vi "_emi_Loop Control single.vi"(0 "Loop ID in":u16, 7 "Enable":bool, 11 "error in (no error)":errorcluster) -> (4 "Loop ID out":u16, 15 "error out":errorcluster)   [LabVIEW 2011]
uses:
  _emi_Loop control int action.ctl
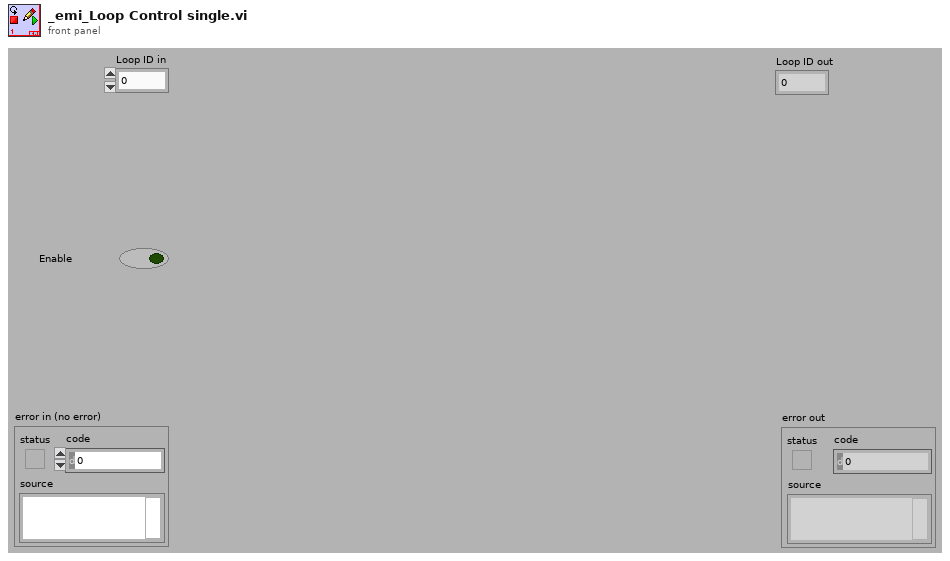
[diagram p1: front panel]
types:
  T1 = typedef "_emi_Loop control int action.ctl" = enum16{"Init index", "Get index", "Set index", "Get Size"}
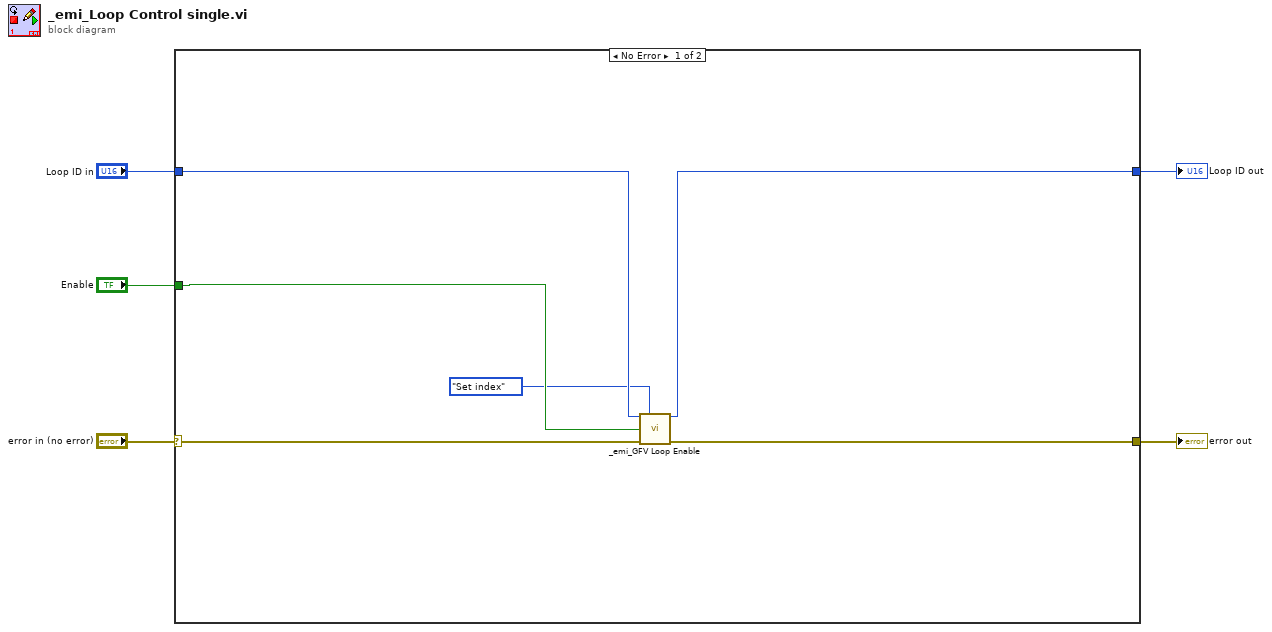
[diagram p0: block diagram]
diagram:
  n1 = case shown="No Error" "error in (no error)" {
    selector: "error in (no error)" -> [w11 w13]
    tunnel: [w10 w13] -> w4
    tunnel: [w8 w12] -> w3
    tunnel: "Loop ID in" -> [w9 w12]
    tunnel: "Enable" -> [w7 _]
    frame No Error {
      n2 = call "_emi_GFV Loop Enable.vi"("Loop Index/Numb"=w9, "Action(Get Index)"=_emi_Loop_control_int_action."Set index", "Loop enable In(T)"=w7, "error in (no error)"=w11) -> ("Index out"=w8:u16, "error out"=w10:errorcluster)  [unwired: 8 in, 2 out]
    }
    frame Error {
    }
  }
  "error out" <- w4
  "Loop ID out" <- w3
